vi "module-05-edge-trigger.vi"() -> ()   [LabVIEW 2019]
uses:
  samples-common-library/Ctrl_Training_Library_Protected/CtrlTrainingLibary_Protected.lvlib
panel:
  in  "Tab Control":enum32{"Ctrl Panel", "Logic"}(tab)
  in  "Switch\nInput":bool
  out "input":bool
  out "On edge":bool
  out "Off Edge":bool
  out "Change Edge":bool
  in  "Scan\nFast / Slow":bool
  out "Scan Time -  Seconds":dbl
  out "Digital State Chart":cluster{dbl, dbl, dbl, dbl, dbl, dbl}(graph)
  # "EDGE TRIGGER TEST"
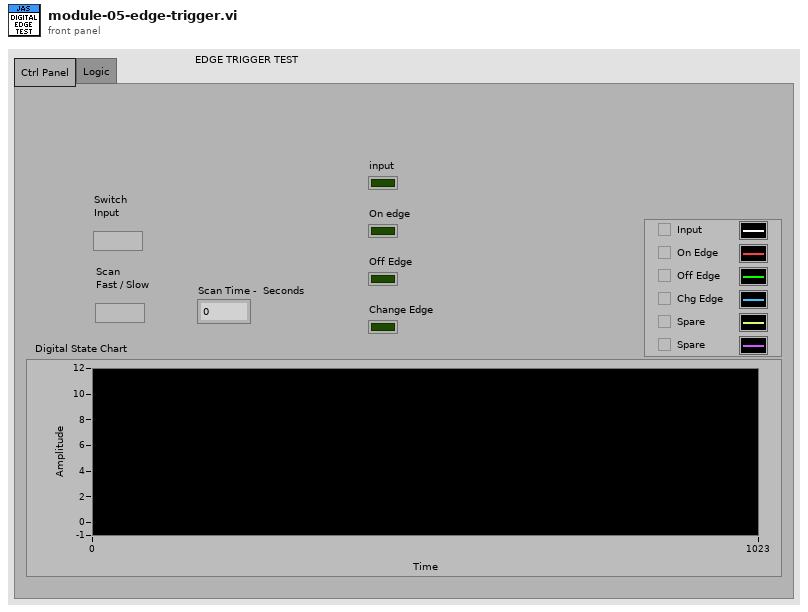
[diagram p1: front panel]
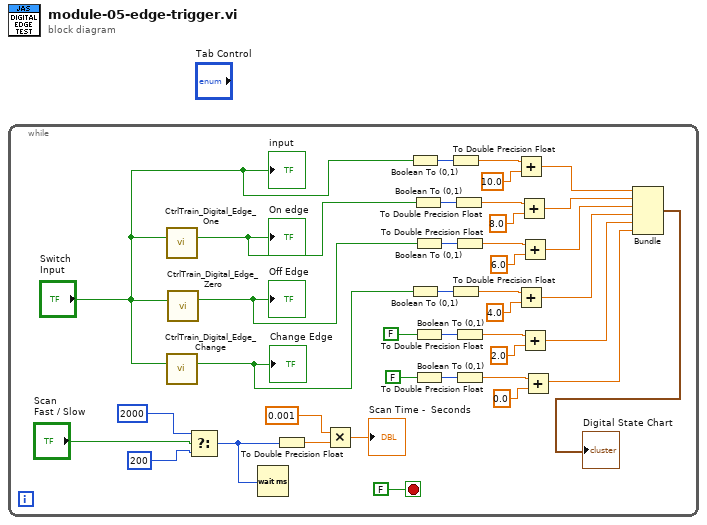
[diagram p0: block diagram]
diagram:
  n1 = while {
    stop <- FALSE stop-if-true
    n2 = call "CtrlTrain_Digital_Edge_One.vi"("Input"="Switch\nInput") -> ("Output"=w4:bool)  [unwired: 14 in]
    "On edge" <- w4
    n3 = call "CtrlTrain_Digital_Edge_Change.vi"("Input"="Switch\nInput") -> ("Output"=w5:bool)  [unwired: 14 in]
    "Change Edge" <- w5
    n4 = call "CtrlTrain_Digital_Edge_Zero.vi"("Input"="Switch\nInput") -> ("Output"=w6:bool)  [unwired: 14 in]
    "Off Edge" <- w6
    n5 = Select(t=u32 2000 ("milliseconds to wait"), s="Scan\nFast / Slow", f=u32 200 ("milliseconds to wait")) -> (s? t:f=w35:u32)
    n6 = Wait (ms)(milliseconds to wait=w35) -> ()  [unwired: 1 out]
    n7 = To Double Precision Float(number=w35) -> (double precision float=w33:dbl)
    n8 = Multiply(x=0.001, y=w33) -> (x*y=→"Scan Time -  Seconds":dbl)
    n9 = Boolean To (0,1)(Boolean="Switch\nInput") -> (0, 1=w14:i16)
    n10 = Boolean To (0,1)(Boolean=w5) -> (0, 1=w15:i16)
    n11 = Boolean To (0,1)(Boolean=w4) -> (0, 1=w17:i16)
    n12 = Boolean To (0,1)(Boolean=w6) -> (0, 1=w19:i16)
    n13 = Boolean To (0,1)(Boolean=FALSE) -> (0, 1=w21:i16)
    n14 = Boolean To (0,1)(Boolean=FALSE) -> (0, 1=w23:i16)
    n15 = To Double Precision Float(number=w14) -> (double precision float=w30:dbl)
    n16 = To Double Precision Float(number=w15) -> (double precision float=w16:dbl)
    n17 = To Double Precision Float(number=w17) -> (double precision float=w18:dbl)
    n18 = To Double Precision Float(number=w19) -> (double precision float=w20:dbl)
    n19 = To Double Precision Float(number=w21) -> (double precision float=w22:dbl)
    n20 = To Double Precision Float(number=w23) -> (double precision float=w24:dbl)
    n21 = Add(x=w30, y=10.0) -> (x+y=w31:dbl)
    n22 = Add(x=w16, y=4.0) -> (x+y=w29:dbl)
    n23 = Add(x=w18, y=8.0) -> (x+y=w27:dbl)
    n24 = Add(x=w20, y=6.0) -> (x+y=w28:dbl)
    n25 = Add(x=w22, y=2.0) -> (x+y=w25:dbl)
    n26 = Add(x=w24, y=0.0) -> (x+y=w26:dbl)
    n27 = Bundle(w31, w27, w28, w29, w25, w26) -> (→"Digital State Chart":cluster{dbl, dbl, dbl, dbl, dbl, dbl})  [unwired: 1 in]
    "input" <- "Switch\nInput"
  }
